vi "Translation Chart View.vi"(10 "User Events in":refnum<class "User Events.lvclass">) -> ()   [LabVIEW 2016, in "FAMT Views.lvlib"]
uses:
  FAMT Views.lvlib
  User Events/User Events.lvclass
  User Events/User Events.lvclass/User Events.ctl
  Typedefs/StateTypes.ctl
  Typedefs/FAMT Typedefs.lvlib
panel:
  out "Chart":T1(graph)
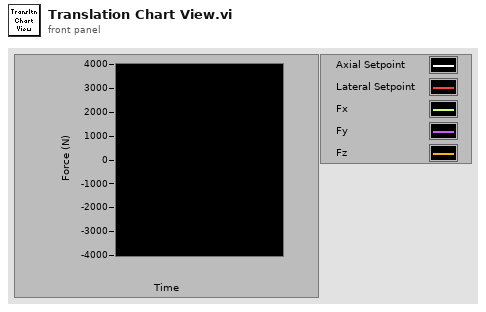
[diagram p1: front panel]
types:
  T1 = cluster{"Axial Demand":dbl, "Lateral Demand":dbl, dbl, dbl, dbl}
  T2 = typedef "FAMT Typedefs.lvlib/Publish Data Events.ctl" = cluster{"State":refnum<user-event>, "ErrorCode":refnum<user-event>, "Scan Progress":refnum<user-event>, "All Test Status":refnum<user-event>}
  T3 = cluster{"Event Registration Refnum":refnum<event-registration>, "Event Registration Refnum":refnum<event-registration>}
  T4 = typedef "FAMT Typedefs.lvlib/StateTypes.ctl" = enum16{"Offline State", "Fault State", "Standby State", "Disabled State", "Enabled State", "Wait For User Input State", "Test Actuator State"}
  T5 = cluster{"Axial Force":dbl, "Axial Force":dbl, "Fx":dbl, "Fy":dbl, "Fz":dbl}
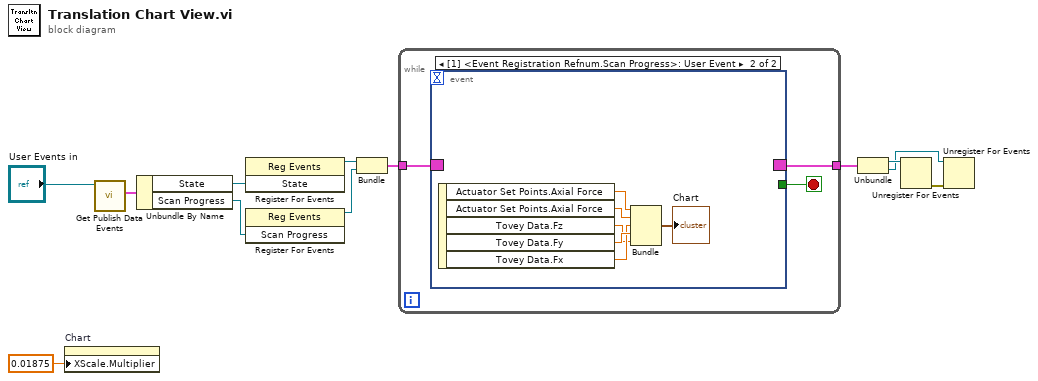
[diagram p0: block diagram]
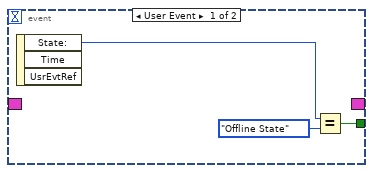
[diagram p2: hidden frame]
diagram:
  n1 = property on="Chart" class="WFChart (strict)"("XScale.Multiplier"=0.01875 ("y")) -> ()  [unwired: 2 in, 2 out]
  n2 = call "Get Publish Data Events.vi"("UserEvents in"="User Events in") -> ("Publish Data Events"=w9:T2)  [unwired: 9 in, 1 out]
  n3 = Unbundle By Name(w9) -> ("State"=w10:refnum<user-event>, "Scan Progress"=w8:refnum<user-event>)
  n4 = register-events(w10) -> (reference out=w12:refnum<event-registration>)  [unwired: 2 in, 1 out]
  n5 = register-events(w8) -> (reference out=w11:refnum<event-registration>)  [unwired: 2 in, 1 out]
  n6 = Bundle("Event Registration Refnum"=w12, "Event Registration Refnum"=w11) -> (w4:T3)  [unwired: 1 in]
  n7 = while {
    tunnel: w4 -> [w15]
    tunnel: [w14] -> w3
    stop <- w13 stop-if-true
    n8 = event shown="[1] <Event Registration Refnum.Scan Progress>: User Event" {
      selector: w15 -> [_ _]
      dyn-events: [_ _] -> w14
      timeout: _ -> [_ _]
      tunnel: [w17 _] -> w13
      event User Event {
        n9 = event-data() -> ("State:"=w16:T4)  [unwired: 1 in, 2 out]
        n10 = Equal?(x=w16, y=StateTypes."Offline State") -> (x = y?=w17:bool)
      }
      event User Event {
        n11 = event-data() -> ("Actuator Set Points.Axial Force"=w24:dbl, "Actuator Set Points.Axial Force"=w22:dbl, "Tovey Data.Fz"=w19:dbl, "Tovey Data.Fy"=w23:dbl, "Tovey Data.Fx"=w20:dbl)  [unwired: 1 in]
        n12 = Bundle("Axial Force"=w24, "Axial Force"=w22, "Fx"=w20, "Fy"=w23, "Fz"=w19) -> (→"Chart":T5)  [unwired: 1 in]
      }
    }
  }
  n13 = Unbundle(w3) -> ("Event Registration Refnum"=w7:refnum<event-registration>, "Event Registration Refnum"=w6:refnum<event-registration>)
  n14 = Unregister For Events(event registration refnum=w7) -> (error out=w5:errorcluster)  [unwired: 1 in]
  n15 = Unregister For Events(event registration refnum=w6, error in=w5) -> ()  [unwired: 1 out]
